vi "Obtain Request Events.vi"(8 "error in (no error)":errorcluster, 10 "Create New? (F)":bool) -> (0 "error out":errorcluster, 2 "Panther Dashboard Request Events":T1)   [LabVIEW 2019, in "Panther Dashboard.lvlib"]
doc: "This VI Obtains/Creates the Requests events that will be used for other modules to communicate with the module that owns this VI. These Requests events will be accessed only via Public API methods for this module.\n\n<b>NOTE</b>: The contents of this VI are automatically generated and modified by the <b>Tools > Delacor > DQMH</b> utilities. Consider using those utilities instead of making your own modifications to this VI.\n_____\nBased on DQMH Project Template 6.1.0.94."
uses:
  Panther Dashboard.lvlib
  Request Events--cluster.ctl
  Stop Argument--cluster.ctl
  Show Panel Argument--cluster.ctl
  Hide Panel Argument--cluster.ctl
  Get Module Execution Status Argument--cluster.ctl
  Show Diagram Argument--cluster.ctl
  Scan DQMH Modules Argument--cluster.ctl
  Tree DQMH Selection Argument--cluster.ctl
  Open Module API Tester Argument--cluster.ctl
  Execute Default Event Request Argument--cluster.ctl
  Expand Results Argument--cluster.ctl
panel:
  # "NOTE: The contents of this VI are automatically generated and modified by the Tools > Delacor > DQMH utilities. Consider using those utilities instead of making your own modifications to this VI."
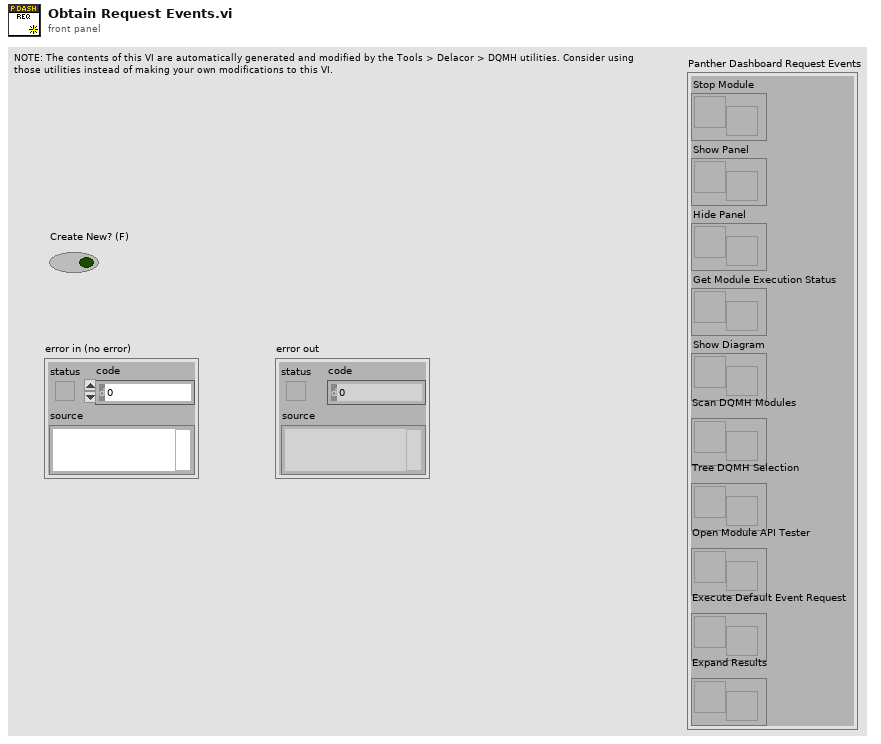
[diagram p1: front panel]
types:
  T1 = typedef "Panther Dashboard.lvlib/Request Events--cluster.ctl" = cluster{"Stop Module":refnum<user-event>, "Show Panel":refnum<user-event>, "Hide Panel":refnum<user-event>, "Get Module Execution Status":refnum<user-event>, "Show Diagram":refnum<user-event>, "Scan DQMH Modules":refnum<user-event>, "Tree DQMH Selection":refnum<user-event>, "Open Module API Tester":refnum<user-event>, "Execute Default Event Request":refnum<user-event>, "Expand Results":refnum<user-event>}
  T2 = typedef "Panther Dashboard.lvlib/Expand Results Argument--cluster.ctl" = cluster{"Expand?":bool}
  T3 = typedef "Panther Dashboard.lvlib/Execute Default Event Request Argument--cluster.ctl" = cluster{"Event Name":string}
  T4 = typedef "Panther Dashboard.lvlib/Open Module API Tester Argument--cluster.ctl" = cluster{"Boolean":bool}
  T5 = typedef "Panther Dashboard.lvlib/Tree DQMH Selection Argument--cluster.ctl" = cluster{"Tree DQMH Sel":string}
  T6 = typedef "Panther Dashboard.lvlib/Scan DQMH Modules Argument--cluster.ctl" = cluster{"Include Dependencies":bool, "Project":string}
  T7 = typedef "Panther Dashboard.lvlib/Hide Panel Argument--cluster.ctl" = cluster{"Hide Panel?":bool}
  T8 = typedef "Panther Dashboard.lvlib/Show Panel Argument--cluster.ctl" = cluster{"Show Panel?":bool}
  T9 = typedef "Panther Dashboard.lvlib/Show Diagram Argument--cluster.ctl" = cluster{"Debug?":bool}
  T10 = typedef "Panther Dashboard.lvlib/Get Module Execution Status Argument--cluster.ctl" = cluster{"Running?":bool}
  T11 = typedef "Panther Dashboard.lvlib/Stop Argument--cluster.ctl" = cluster{"Origin":string, "Exit via Stop Module Req?":bool, "Wait for Module to stop?":bool}
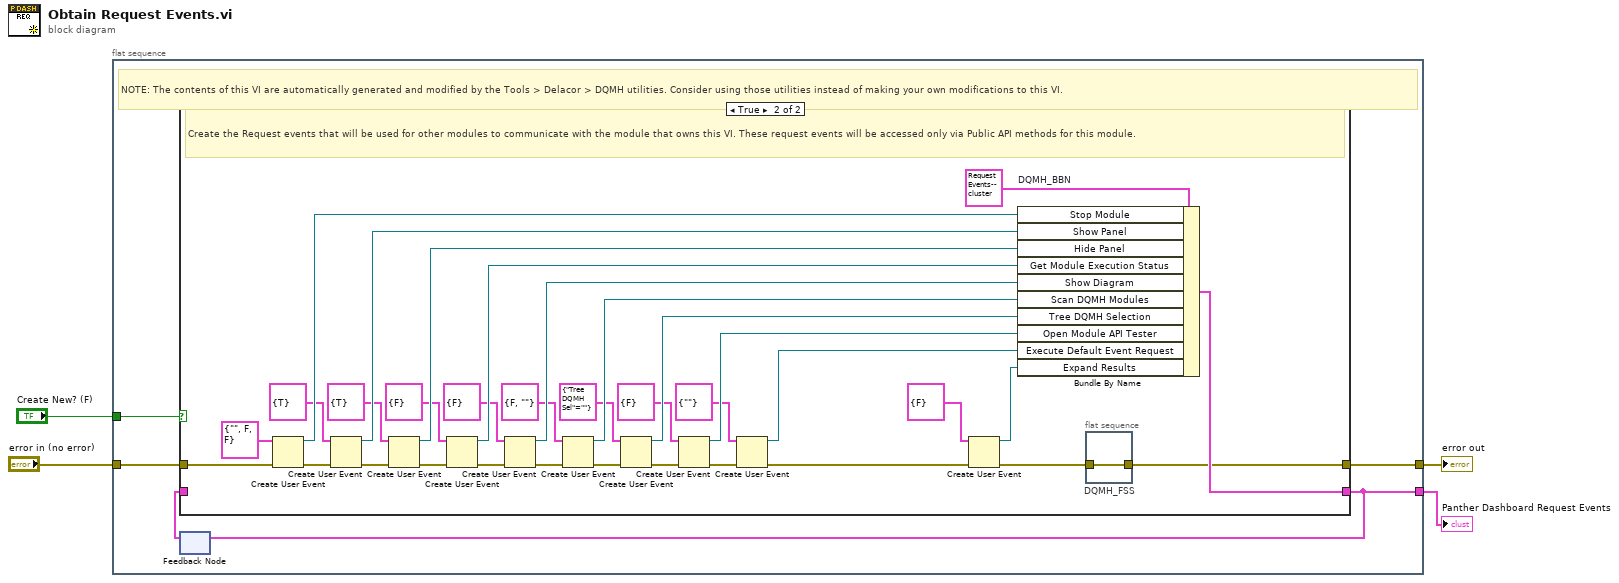
[diagram p0: block diagram]
diagram:
  n1 = flat-sequence {
    tunnel: [w9] -> w4
    tunnel: "error in (no error)" -> [w8]
    tunnel: [w6] -> w2
    tunnel: "Create New? (F)" -> [w5]
    frame #0 {
      # "NOTE: The contents of this VI are automatically generated and modified by the Tools > Delacor > DQMH utilities. Consider using those utilities instead of making your own modifications to this VI."
      n2 = feedback #1() -> (w7:T1)  [unwired: 1 in]
      n3 = case shown="True" w5 {
        tunnel: [w10 w35] -> w9
        tunnel: w8 -> [w10 w45]
        tunnel: [w11 w42] -> w6
        tunnel: w7 -> [w11 _]
        frame False {
          # "Obtain the Request events that were created in a previous call to this VI."
        }
        frame True {
          # "Create the Request events that will be used for other modules to communicate with the module that owns this VI. These request events will be accessed only via Public API methods for this module."
          n4 = Create User Event(user event datatype=T11 {"Origin"="", "Exit via Stop Module Req?"=FALSE, "Wait for Module to stop?"=FALSE} ("Stop Argument"), error in=w45) -> (user event=w43:refnum<user-event>, error out=w40:errorcluster)
          n5 = Create User Event(user event datatype=T8 {"Show Panel?"=TRUE} ("Show Panel Argument"), error in=w40) -> (user event=w39:refnum<user-event>, error out=w38:errorcluster)
          n6 = Create User Event(user event datatype=T7 {"Hide Panel?"=TRUE} ("Hide Panel Argument"), error in=w38) -> (user event=w37:refnum<user-event>, error out=w36:errorcluster)
          n7 = Create User Event(user event datatype=T10 {"Running?"=FALSE} ("Get Module Execution Status Argument"), error in=w36) -> (user event=w33:refnum<user-event>, error out=w34:errorcluster)
          n8 = Create User Event(user event datatype=T9 {"Debug?"=FALSE} ("Show Diagram Argument"), error in=w34) -> (user event=w30:refnum<user-event>, error out=w31:errorcluster)
          n9 = Create User Event(user event datatype=T6 {"Include Dependencies"=FALSE, "Project"=""} ("Scan DQMH Modules Argument"), error in=w31) -> (user event=w25:refnum<user-event>, error out=w26:errorcluster)
          n10 = Create User Event(user event datatype=T5 {"Tree DQMH Sel"=""} ("Tree DQMH Selection Argument"), error in=w26) -> (user event=w22:refnum<user-event>, error out=w23:errorcluster)
          n11 = Create User Event(user event datatype=T4 {"Boolean"=FALSE} ("Open Module API Tester Argument"), error in=w23) -> (user event=w19:refnum<user-event>, error out=w20:errorcluster)
          n12 = Create User Event(user event datatype=T3 {"Event Name"=""} ("Execute Default Event Request Argument"), error in=w20) -> (user event=w16:refnum<user-event>, error out=w17:errorcluster)
          n13 = Create User Event(user event datatype=T2 {"Expand?"=FALSE} ("Expand or Close Argument"), error in=w17) -> (user event=w13:refnum<user-event>, error out=w14:errorcluster)
          n14 = Bundle By Name "DQMH_BBN"(cluster=T1 {"Stop Module"=refnum, "Show Panel"=refnum, "Hide Panel"=refnum, "Get Module Execution Status"=refnum, "Show Diagram"=refnum, "Scan DQMH Modules"=refnum, "Tree DQMH Selection"=refnum, "Open Module API Tester"=refnum, "Execute Default Event Request"=refnum, "Expand Results"=refnum} ("output cluster"), "Stop Module"=w43, "Show Panel"=w39, "Hide Panel"=w37, "Get Module Execution Status"=w33, "Show Diagram"=w30, "Scan DQMH Modules"=w25, "Tree DQMH Selection"=w22, "Open Module API Tester"=w19, "Execute Default Event Request"=w16, "Expand Results"=w13) -> (w42:T1)
          n15 = flat-sequence "DQMH_FSS" {
            tunnel: w14 -> [w46]
            tunnel: [w46] -> w35
            frame #0 {
            }
          }
        }
      }
      n16 = feedback-in #1(w6) -> ()
    }
  }
  "Panther Dashboard Request Events" <- w2
  "error out" <- w4
